vi "TimeIntToTimeRec.vi"(1 "Time Int":u32) -> (0 "TimeRec":T1)   [LabVIEW 2009]
uses:
  TimeRec.ctl
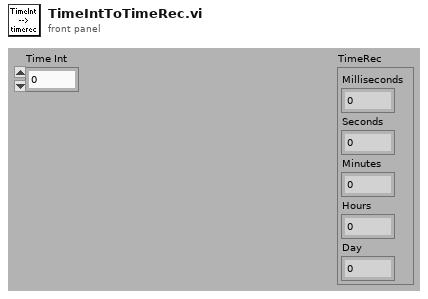
[diagram p1: front panel]
types:
  T1 = typedef "TimeRec.ctl" = cluster{"Milliseconds":u32, "Seconds":u32, "Minutes":u32, "Hours":u32, "Day":u32}
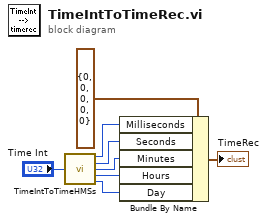
[diagram p0: block diagram]
diagram:
  n1 = call "TimeIntToTimeHMSs.vi"("Time Int"="Time Int") -> ("Milliseconds"=w3:u32, "Seconds"=w5:u32, "Minutes"=w4:u32, "Hours"=w6:u32, "Day"=w7:u32)  [unwired: 10 in]
  n2 = Bundle By Name(cluster=T1 {"Milliseconds"=0, "Seconds"=0, "Minutes"=0, "Hours"=0, "Day"=0} ("TimeRec"), "Milliseconds"=w3, "Seconds"=w5, "Minutes"=w4, "Hours"=w6, "Day"=w7) -> (→"TimeRec":T1)
